vi "Write Spectrum plot.vi"(8 "error in (no error)":errorcluster, 10 "Spectrum plot":cluster{"Array":dbl[], "Array":dbl[]}[](array[cluster]), 11 "Spectrometer Driver in":refnum<class "Spectrometer Driver.lvclass">) -> (0 "error out":errorcluster, 3 "Spectrometer Driver out":refnum<class "Spectrometer Driver.lvclass">)   [LabVIEW 2016, in "Spectrometer Driver.lvclass"]
uses:
  Spectrometer Driver.lvclass
  Spectrometer Driver.lvclass/Spectrometer Driver.ctl
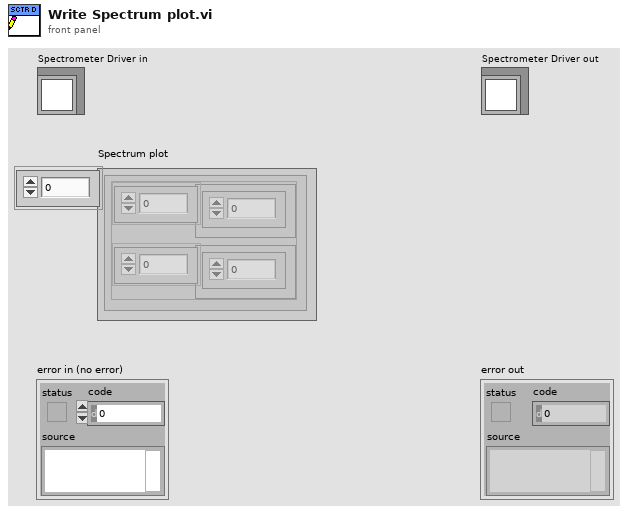
[diagram p1: front panel]
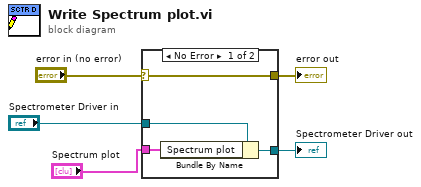
[diagram p0: block diagram]
diagram:
  n1 = case shown="No Error" "error in (no error)" {
    selector: "error in (no error)" -> [w9 w10]
    tunnel: [w9 w10] -> w4
    tunnel: [w7 w11] -> w2
    tunnel: "Spectrometer Driver in" -> [w8 w11]
    tunnel: "Spectrum plot" -> [w6 _]
    frame No Error {
      n2 = Bundle By Name(cluster=w8, "Spectrum plot"=w6) -> (w7:refnum<class "Spectrometer Driver.lvclass">)
    }
    frame Error {
    }
  }
  "error out" <- w4
  "Spectrometer Driver out" <- w2
